vi "I2C WriteRead Data.vi"(5 "Address":T2 format="%02x", 6 "NoStop (F)":bool, 7 "I2C #":T1=-1, 8 "error in (no error)":errorcluster, 9 "Len":u8, 10 "Write Data":string, 11 "VisaComms in":refnum<class "VisaComms.lvclass">) -> (0 "error out":errorcluster, 1 "Read Data":string, 3 "VisaComms out":refnum<class "VisaComms.lvclass">)   [LabVIEW 2020, in "CTI.lvlib" / "VisaComms.lvclass"]
uses:
  VisaComms.lvclass
  I2C Address.ctl
  I2C Number.ctl
  CTI.lvlib
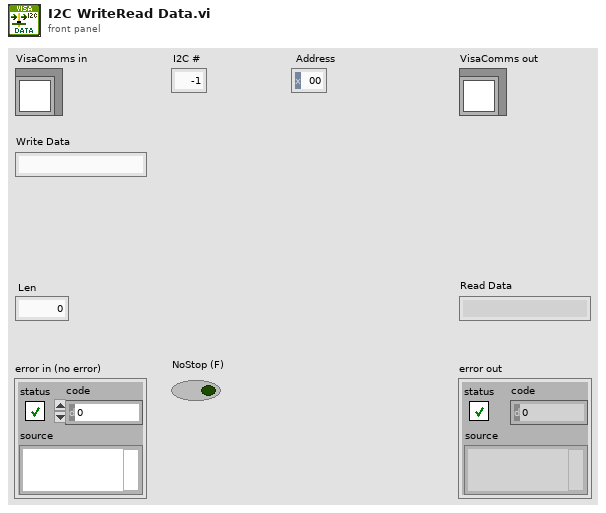
[diagram p1: front panel]
types:
  T1 = typedef "CTI.lvlib/I2C Number.ctl" = i8
  T2 = typedef "CTI.lvlib/I2C Address.ctl" = u8
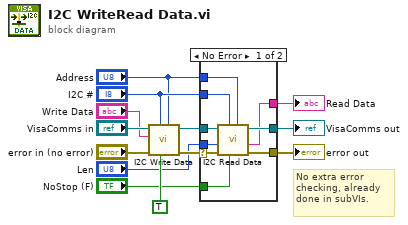
[diagram p0: block diagram]
diagram:
  # "No extra error checking, already done in subVIs."
  n1 = call-dynamic "I2C Write Data.vi"("Address"="Address", "NoStop (F)"=TRUE, "I2C #"="I2C #", "error in (no error)"="error in (no error)", "Data"="Write Data", "VisaComms in"="VisaComms in") -> ("error out"=w12:errorcluster, "VisaComms out"=w7:refnum<class "VisaComms.lvclass">)  [unwired: 4 in]
  n2 = case shown="No Error" w12 {
    selector: w12 -> [w22 w23]
    tunnel: [w21 w23] -> w8
    tunnel: w7 -> [w20 w24]
    tunnel: [w19 w24] -> w6
    tunnel: "Len" -> [w18 _]
    tunnel: "NoStop (F)" -> [w17 _]
    tunnel: "I2C #" -> [w16 _]
    tunnel: "Address" -> [w15 _]
    tunnel: [w14 _] -> w1
    frame No Error {
      n3 = call-dynamic "I2C Read Data.vi"("Address"=w15, "NoStop (F)"=w17, "I2C #"=w16, "error in (no error)"=w22, "Len"=w18, "VisaComms in"=w20) -> ("error out"=w21:errorcluster, "Data"=w14:string, "VisaComms out"=w19:refnum<class "VisaComms.lvclass">)  [unwired: 3 in]
    }
    frame Error {
    }
  }
  "error out" <- w8
  "VisaComms out" <- w6
  "Read Data" <- w1
